vi "1 axis move.vi"(2 "Deceleration":bool, 4 "RESET":bool, 5 "Stop":bool, 6 "Accelaration":bool, 7 "error in (no error)":errorcluster, 8 "A axis":i32, 9 "Comport":refnum<visa-resource-name>) -> (3 "A out":dbl)   [LabVIEW 2020]
uses:
  <vilib>/Instr/_visa.llb/VISA Configure Serial Port (Instr).vi
  GlobalValue.vi
panel:
  # "COMPORT"
  # "To Move"
  # "Moved"
  # "Microns"
  # "Microns"
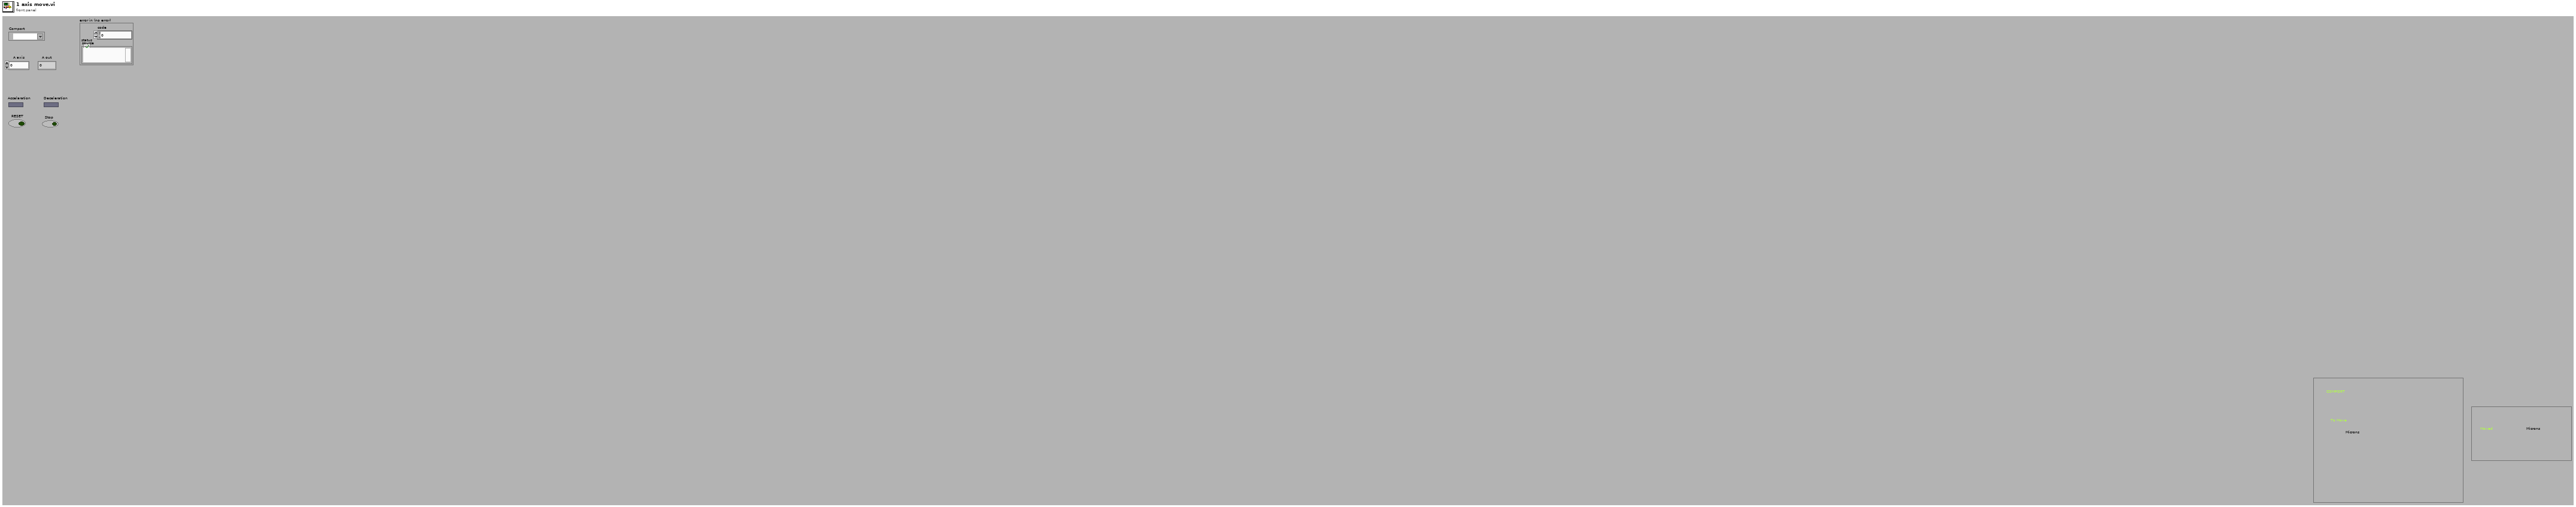
[diagram p1: front panel]
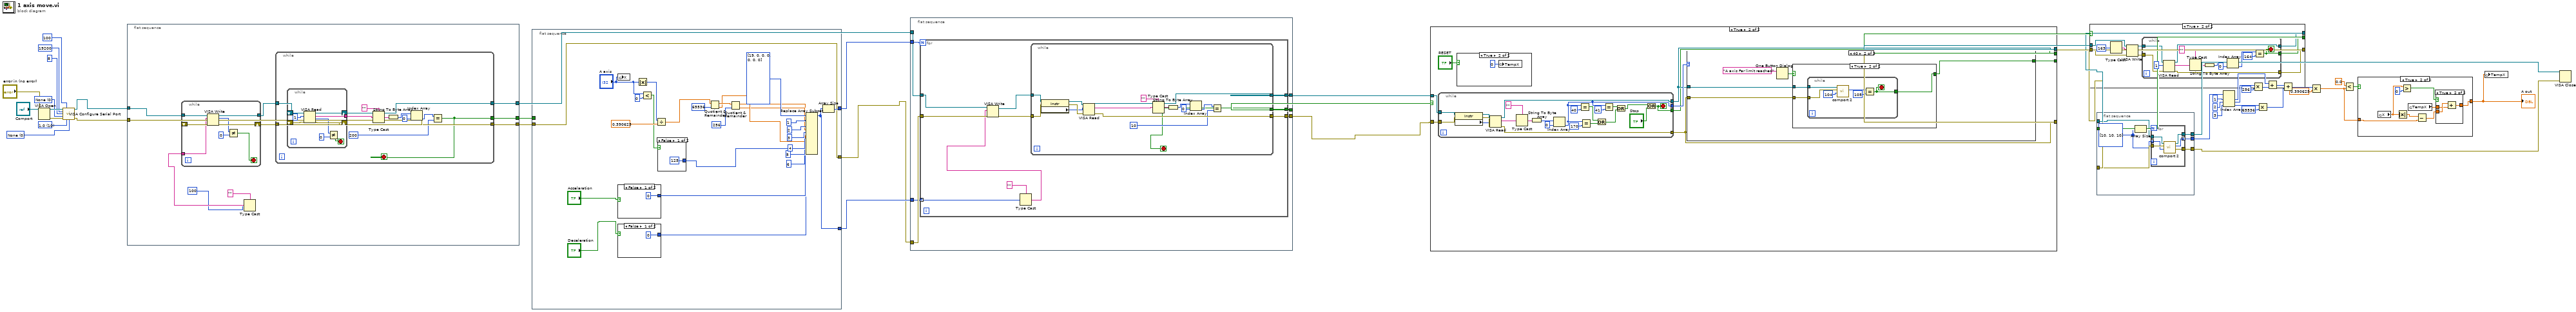
[diagram p0: block diagram]
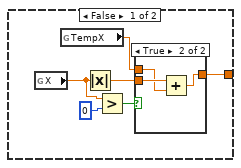
[diagram p2: hidden frame]
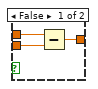
[diagram p3: hidden frame]
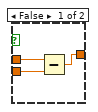
[diagram p4: hidden frame]
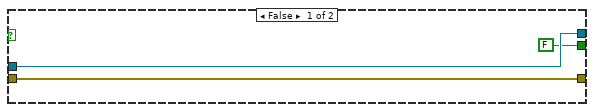
[diagram p5: hidden frame]
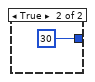
[diagram p6: hidden frame]
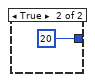
[diagram p7: hidden frame]
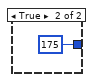
[diagram p8: hidden frame]
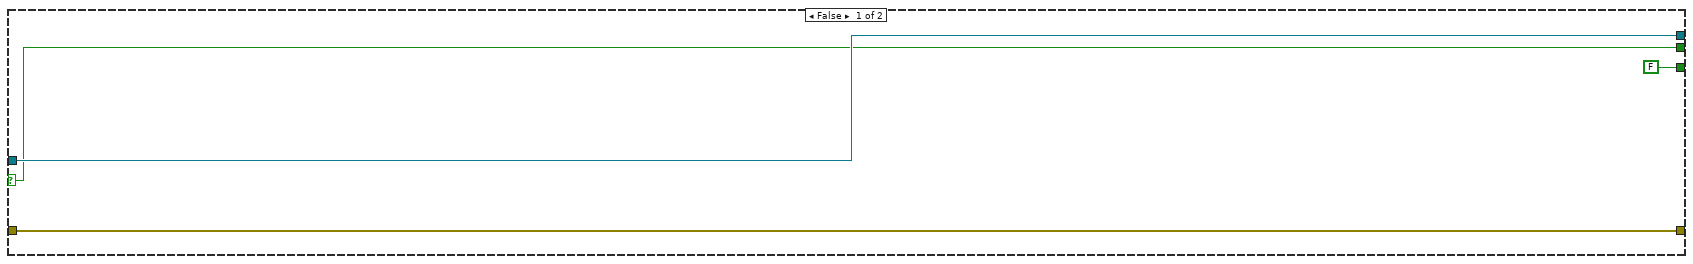
[diagram p9: hidden frame]
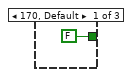
[diagram p11: hidden frame]
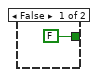
[diagram p12: hidden frame]
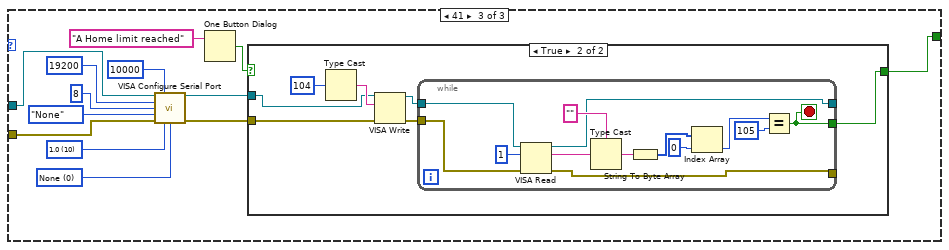
[diagram p13: hidden frame]
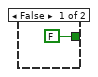
[diagram p14: hidden frame]
diagram:
  w42 = u16 0 items=["None"=0, "XON/XOFF"=1, "RTS/CTS"=2, "DTR/DSR"=4] ("flow control")
  w41 = u16 10 items=["1.0"=10, "1.5"=15, "2.0"=20] ("stop bits")
  w40 = u16 0 items=["None", "Odd", "Even", "Mark", "Space"] ("parity")
  n1 = VISA Open(error in (no error)="error in (no error)", VISA resource name="Comport") -> (VISA resource name=w45:refnum<visa-resource-name>, error out=w46:errorcluster)  [unwired: 3 in]
  n2 = call-poly "VISA Configure Serial Port"("VISA resource name"=w45, "timeout (10sec)"=u32 100, "baud rate (9600)"=u32 19200 ("baud rate"), "data bits (8)"=u16 8 ("data bits"), "parity (0:none)"=w40, "error in (no error)"=w46, "stop bits (10: 1 bit)"=w41, "flow control (0:none)"=w42) -> ("VISA resource name out"=w37:refnum<visa-resource-name>, "error out"=w36:errorcluster)  [unwired: 1 in, 5 out]
  n3 = flat-sequence {
    tunnel: w37 -> [w57]
    tunnel: w36 -> [w56]
    tunnel: [w55] -> w34
    tunnel: [w54] -> w3
    tunnel: [w48] -> w4
    frame #0 {
      n4 = Type Cast(type="", x=u8 100) -> (*(type *) &x=w52:string)
      n5 = while {
        tunnel: w52 -> [w65]
        shift-right: [w61] -> w49
        shift-left: w56 -> [w63]
        tunnel: w57 -> [w64]
        tunnel: [w62] -> w50
        stop <- w58 stop-if-true
        n6 = VISA Write(VISA resource name=w64, write buffer=w65, error in (no error)=w63) -> (VISA resource name out=w62:refnum<visa-resource-name>, return count=w60:u32, error out=w61:errorcluster)
        n7 = Not Equal?(x=w60, y=u32 0) -> (x != y?=w58:bool)
      }
      n8 = while {
        tunnel: w49 -> [w76]
        tunnel: [w74] -> w54
        tunnel: w50 -> [w77]
        tunnel: [w75] -> w55
        tunnel: [w69] -> w48
        stop <- w69 stop-if-true
        n9 = while {
          tunnel: [w81] -> w68
          shift-right: [w84] -> w75
          shift-left: w77 -> [w86]
          shift-right: [w83] -> w74
          shift-left: w76 -> [w85]
          stop <- w78 stop-if-true
          n10 = VISA Read(VISA resource name=w86, byte count=u32 1, error in (no error)=w85) -> (VISA resource name out=w84:refnum<visa-resource-name>, read buffer=w81:string, return count=w79:u32, error out=w83:errorcluster)
          n11 = Not Equal?(x=w79, y=u32 0) -> (x != y?=w78:bool)
        }
        n12 = Type Cast(type="", x=w68) -> (*(type *) &x=w66:string)
        n13 = String To Byte Array(string=w66) -> (unsigned byte array=w73:u8[])
        n14 = Index Array(array=w73, index=0) -> (element=w71:u8)
        n15 = Equal?(x=w71, y=u8 200) -> (x = y?=w69:bool)
      }
    }
  }
  n16 = flat-sequence {
    tunnel: [w107] -> w35
    tunnel: [w106] -> w33
    tunnel: w4 -> [_]
    tunnel: w3 -> [w94]
    tunnel: [w94] -> w2
    frame #0 {
      n17 = global write "GlobalValue.vi" "X"("A axis") -> ()
      n18 = case shown="False" "Accelaration" {
        tunnel: [0 20] -> w101
        frame False {
        }
        frame True {
        }
      }
      n19 = case shown="False" "Deceleration" {
        tunnel: [0 30] -> w99
        frame False {
        }
        frame True {
        }
      }
      n20 = Absolute Value(x="A axis") -> (abs(x)=w109:i32)
      n21 = Less?(x="A axis", y=0) -> (x < y?=w111:bool)
      n22 = Divide(x=w109, y=0.390625) -> (x/y=w93:dbl)
      n23 = case shown="False" w111 {
        tunnel: [u16 125 u16 175] -> w103
        frame False {
        }
        frame True {
        }
      }
      n24 = Quotient & Remainder(x=w93, y=65536) -> (x-y*floor(x/y)=w91:dbl, floor(x/y)=w89:dbl)
      n25 = Quotient & Remainder(x=w91, y=256) -> (x-y*floor(x/y)=w87:dbl, floor(x/y)=w88:dbl)
      n26 = Replace Array Subset(array=u8[] [19, 0, 0, 0, 0, 0, 0], new element #1=w87, index #1=1 ("index"), new element #2=w88, index #2=2 ("index"), new element #3=w89, index #3=3 ("index"), new element #4=w103, index #4=4 ("index"), new element #5=w101, index #5=5 ("index"), new element #6=w99, index #6=6 ("index")) -> (w106:u8[])
      n27 = Array Size(array=w106) -> (size(s)=w107:i32)
    }
  }
  n28 = flat-sequence {
    tunnel: w35 -> [w126]
    tunnel: w34 -> [w125]
    tunnel: w2 -> [w124]
    tunnel: w33 -> [w123]
    tunnel: [w122] -> w32
    tunnel: [w121] -> w1
    tunnel: [w120] -> w31
    frame #0 {
      n29 = for {
        N: w126 -> [_]
        tunnel: [w131] -> w120
        tunnel: w125 -> [w135]
        tunnel: [w133] -> w122
        tunnel: w124 -> [w134]
        tunnel: [w132] -> w121
        tunnel: w123 -> [w128] mode=indexing
        n30 = Type Cast(type="", x=w128) -> (*(type *) &x=w127:string)
        n31 = VISA Write(VISA resource name=w135, write buffer=w127, error in (no error)=w134) -> (VISA resource name out=w130:refnum<visa-resource-name>, error out=w129:errorcluster)  [unwired: 1 out]
        n32 = while {
          tunnel: w129 -> [w140]
          tunnel: [w150] -> w132
          tunnel: w130 -> [w141]
          tunnel: [w151] -> w133
          tunnel: [w145] -> w131
          stop <- w145 stop-if-true
          n33 = property class="Instr"(reference=w141, error in=w140) -> (reference out=w139:refnum<visa-resource-name>, error out=w138:errorcluster, "Serial Settings:Number of Bytes at Serial Port"=w137:u32)
          n34 = VISA Read(VISA resource name=w139, byte count=w137, error in (no error)=w138) -> (VISA resource name out=w151:refnum<visa-resource-name>, read buffer=w144:string, error out=w150:errorcluster)  [unwired: 1 out]
          n35 = Type Cast(type="", x=w144) -> (*(type *) &x=w142:string)
          n36 = String To Byte Array(string=w142) -> (unsigned byte array=w149:u8[])
          n37 = Index Array(array=w149, index=0) -> (element=w147:u8)
          n38 = Equal?(x=w147, y=u8 10) -> (x = y?=w145:bool)
        }
      }
    }
  }
  n39 = case shown="True" w31 {
    selector: w31 -> [w152 _]
    tunnel: w32 -> [w155 w160]
    tunnel: w1 -> [w154 w162]
    tunnel: [w155 w159] -> w30
    tunnel: [w154 w158] -> w28
    tunnel: [w152 w156] -> w29
    tunnel: [FALSE w157] -> _
    frame False {
    }
    frame True {
      n40 = while {
        tunnel: w162 -> [w167]
        tunnel: [w173] -> w159
        tunnel: [w176] -> w158
        tunnel: [w175] -> w156
        tunnel: [w172] -> w161
        tunnel: w160 -> [w168]
        stop <- w175 stop-if-true
        n41 = property class="Instr"(reference=w168, error in=w167) -> (reference out=w166:refnum<visa-resource-name>, error out=w165:errorcluster, "Serial Settings:Number of Bytes at Serial Port"=w164:u32)
        n42 = VISA Read(VISA resource name=w166, byte count=w164, error in (no error)=w165) -> (VISA resource name out=w173:refnum<visa-resource-name>, read buffer=w185:string, error out=w176:errorcluster)  [unwired: 1 out]
        n43 = Type Cast(type="", x=w185) -> (*(type *) &x=w186:string)
        n44 = String To Byte Array(string=w186) -> (unsigned byte array=w184:u8[])
        n45 = Index Array(array=w184, index=0) -> (element=w172:u8)
        n46 = Equal?(x=w172, y=u8 40) -> (x = y?=w171:bool)
        n47 = Equal?(x=w172, y=u8 170) -> (x = y?=w174:bool)
        n48 = Or(x=w171, y=w174) -> (x .or. y?=w170:bool)
        n49 = Equal?(x=w172, y=u8 41) -> (x = y?=w179:bool)
        n50 = Or(x=w179, y=w170) -> (x .or. y?=w169:bool)
        n51 = Or(x=w169, y="Stop") -> (x .or. y?=w175:bool)
      }
      n52 = case shown="True" "RESET" {
        frame False {
        }
        frame True {
          n53 = global write "GlobalValue.vi" "TempX"(0) -> ()
        }
      }
      n54 = case shown="40" w161 {
        tunnel: w159 -> [_ w190 w213]
        tunnel: w158 -> [_ w191 w210]
        tunnel: [FALSE w189 w214] -> w157
        frame 170, Default {
        }
        frame 40 {
          n55 = One Button Dialog(message="A axis Far limit reached") -> (true=w192:bool)  [unwired: 1 in]
          n56 = case shown="True" w192 {
            tunnel: w191 -> [_ w196]
            tunnel: w190 -> [_ w197]
            tunnel: [FALSE w195] -> w189
            frame False {
            }
            frame True {
              n57 = while {
                tunnel: w197 -> [w203]
                tunnel: w196 -> [w202]
                tunnel: [w198] -> w195
                stop <- w198 stop-if-true
                n58 = call "comport 2.vi"("x"=u8 104, "error in (no error)"=w202, "VISA resource name"=w203) -> ("Numeric"=w200:u8)  [unwired: 6 in, 2 out]
                n59 = Equal?(x=w200, y=u8 105) -> (x = y?=w198:bool)
              }
            }
          }
        }
        frame 41 {
          w205 = u16 0 items=["None", "XON/XOFF", "RTS/CTS", "XON/XOFF & RTS/CTS", "DTR/DSR", "XON/XOFF & DTR/DSR"] ("flow control (0:none)")
          w206 = u16 10 items=["1.0"=10, "1.5"=15, "2.0"=20] ("stop bits (10: 1 bit)")
          n60 = call-poly "VISA Configure Serial Port"("VISA resource name"=w213, "timeout (10sec)"=u32 10000, "baud rate (9600)"=u32 19200, "data bits (8)"=u16 8, "parity (0:none)"=enum16{"None", "Odd", "Even", "Mark", "Space"}."None", "error in (no error)"=w210, "stop bits (10: 1 bit)"=w206, "flow control (0:none)"=w205) -> ("VISA resource name out"=w212:refnum<visa-resource-name>, "error out"=w211:errorcluster)  [unwired: 6 in]
          n61 = One Button Dialog(message="A Home limit reached") -> (true=w215:bool)  [unwired: 1 in]
          n62 = case shown="True" w215 {
            tunnel: w212 -> [_ w221]
            tunnel: w211 -> [_ w220]
            tunnel: [FALSE w218] -> w214
            frame False {
            }
            frame True {
              n63 = Type Cast(x=104) -> (*(type *) &x=w224:string)  [unwired: 1 in]
              n64 = VISA Write(VISA resource name=w221, write buffer=w224, error in (no error)=w220) -> (VISA resource name out=w222:refnum<visa-resource-name>, error out=w223:errorcluster)  [unwired: 1 out]
              n65 = while {
                tunnel: w223 -> [w237]
                tunnel: [w227] -> _
                tunnel: w222 -> [w236]
                tunnel: [w226] -> _
                tunnel: [w225] -> w218
                stop <- w225 stop-if-true
                n66 = VISA Read(VISA resource name=w236, byte count=u32 1, error in (no error)=w237) -> (VISA resource name out=w226:refnum<visa-resource-name>, read buffer=w228:string, error out=w227:errorcluster)  [unwired: 1 out]
                n67 = Type Cast(type="", x=w228) -> (*(type *) &x=w229:string)
                n68 = String To Byte Array(string=w229) -> (unsigned byte array=w233:u8[])
                n69 = Index Array(array=w233, index=0) -> (element=w230:u8)
                n70 = Equal?(x=w230, y=u8 105) -> (x = y?=w225:bool)
              }
            }
          }
        }
      }
    }
  }
  n71 = case shown="True" w29 {
    tunnel: w30 -> [w240 w246]
    tunnel: w28 -> [w239 w245]
    tunnel: [FALSE w244] -> w5
    tunnel: [w240 w242] -> w27
    tunnel: [w239 w243] -> w26
    frame False {
    }
    frame True {
      n72 = Type Cast(x=163) -> (*(type *) &x=w249:string)  [unwired: 1 in]
      n73 = VISA Write(VISA resource name=w246, write buffer=w249, error in (no error)=w245) -> (VISA resource name out=w247:refnum<visa-resource-name>, error out=w248:errorcluster)  [unwired: 1 out]
      n74 = while {
        tunnel: w248 -> [w262]
        tunnel: [w252] -> w243
        tunnel: w247 -> [w261]
        tunnel: [w251] -> w244
        tunnel: [w250] -> w242
        stop <- w251 stop-if-true
        n75 = VISA Read(VISA resource name=w261, byte count=u32 1, error in (no error)=w262) -> (VISA resource name out=w250:refnum<visa-resource-name>, read buffer=w253:string, error out=w252:errorcluster)  [unwired: 1 out]
        n76 = Type Cast(type="", x=w253) -> (*(type *) &x=w254:string)
        n77 = String To Byte Array(string=w254) -> (unsigned byte array=w258:u8[])
        n78 = Index Array(array=w258, index=0) -> (element=w255:u8)
        n79 = Equal?(x=w255, y=u8 164) -> (x = y?=w251:bool)
      }
    }
  }
  n80 = flat-sequence {
    tunnel: w26 -> [w268]
    tunnel: [w266] -> w24
    tunnel: [w267] -> w25
    tunnel: w27 -> [w265]
    tunnel: [w264] -> w23
    tunnel: w5 -> [_]
    frame #0 {
      w263 = u8[] [10, 10, 10]
      n81 = Array Size(array=w263) -> (size(s)=w269:i32)
      n82 = for {
        N: w269 -> [_]
        tunnel: w268 -> [w273]
        tunnel: [w274] -> w267
        tunnel: w265 -> [w275]
        tunnel: [w270] -> w266
        tunnel: [w271] -> w264 mode=indexing
        tunnel: w263 -> [w272] mode=indexing
        n83 = call "comport 2.vi"("x"=w272, "error in (no error)"=w273, "VISA resource name"=w275) -> ("error out"=w270:errorcluster, "Numeric"=w271:u8, "VISA resource name out"=w274:refnum<visa-resource-name>)  [unwired: 6 in]
      }
    }
  }
  n84 = Index Array(array=w23, index #1=1 ("index"), index #2=2 ("index"), index #3=3 ("index")) -> (element #1=w8:u8, element #2=w7:u8, element #3=w6:u8)
  n85 = Multiply(x=w7, y=u16 256) -> (x*y=w18:u16)
  n86 = Multiply(x=w6, y=u32 65536) -> (x*y=w17:u32)
  n87 = Add(x=w8, y=w18) -> (x+y=w16:u16)
  n88 = Add(x=w16, y=w17) -> (x+y=w12:u32)
  n89 = Multiply(x=w12, y=0.390625) -> (x*y=w13:dbl)
  n90 = Less?(x=0.0, y=w13) -> (x < y?=w14:bool)
  n91 = case shown="True" w14 {
    tunnel: w13 -> [_ w295]
    tunnel: [w278 w290] -> w22
    frame False {
      n92 = global read "GlobalValue.vi" "X"() -> (w277:dbl)
      n93 = global read "GlobalValue.vi" "TempX"() -> (w279:dbl)
      n94 = Absolute Value(x=w277) -> (abs(x)=w276:dbl)
      n95 = Greater?(x=w277, y=0) -> (0:w280:bool)
      n96 = case shown="True" w280 {
        tunnel: w276 -> [w283 w287]
        tunnel: w279 -> [w284 w286]
        tunnel: [w282 w285] -> w278
        frame False {
          n97 = Subtract(x=w284, y=w283) -> (x-y=w282:dbl)
        }
        frame True {
          n98 = Add(x=w287, y=w286) -> (x+y=w285:dbl)
        }
      }
    }
    frame True {
      n99 = global read "GlobalValue.vi" "X"() -> (w289:dbl)
      n100 = Absolute Value(x=w289) -> (abs(x)=w288:dbl)
      n101 = Greater?(x=w289, y=0) -> (0:w293:bool)
      n102 = global read "GlobalValue.vi" "TempX"() -> (w291:dbl)
      n103 = Subtract(x=w288, y=w295) -> (x-y=w292:dbl)
      n104 = case shown="True" w293 {
        tunnel: w292 -> [w297 w301]
        tunnel: w291 -> [w298 w300]
        tunnel: [w296 w299] -> w290
        frame False {
          n105 = Subtract(x=w298, y=w297) -> (x-y=w296:dbl)
        }
        frame True {
          n106 = Add(x=w301, y=w300) -> (x+y=w299:dbl)
        }
      }
    }
  }
  "A out" <- w22
  n107 = global write "GlobalValue.vi" "TempX"(w22) -> ()
  n108 = VISA Close(VISA resource name=w25, error in (no error)=w24) -> ()  [unwired: 1 out]
